vi "数组拆分.vi"(10 "拆分大小":i32=1000, 11 "输入数据":string[][](array[string])) -> (3 "输出数组":string[][](array[string]))   [LabVIEW 2016, in "数据传输系统-03.lvlib"]
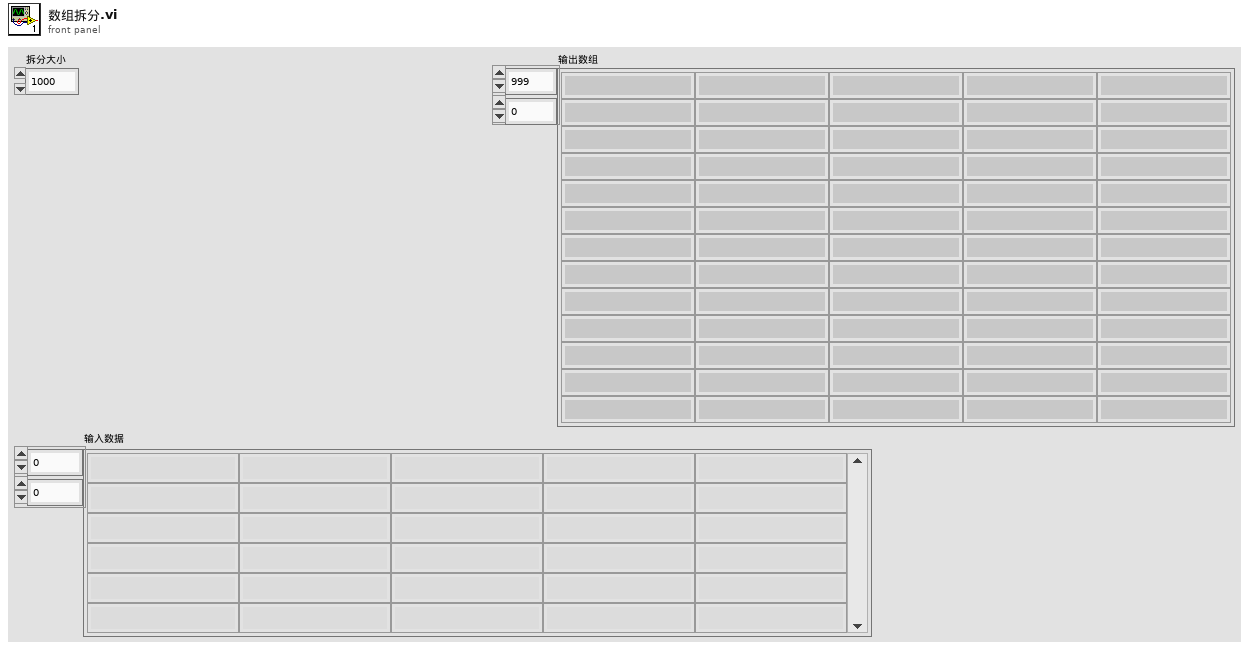
[diagram p1: front panel]
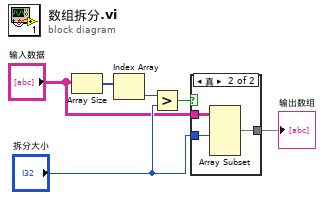
[diagram p0: block diagram]
diagram:
  n1 = Array Size(array="输入数据") -> (size(s)=w6:i32[])
  n2 = Index Array(array=w6) -> (element=w5:i32)  [unwired: 1 in]
  n3 = Greater?(x=w5, y="拆分大小") -> (0:w4:bool)
  n4 = case shown="真" w4 {
    tunnel: "输入数据" -> [w7 w10]
    tunnel: "拆分大小" -> [_ w9]
    tunnel: [w7 w8] -> w1
    frame False {
    }
    frame True {
      n5 = Array Subset(array=w10, length (row)=w9) -> (w8:string[][])  [unwired: 3 in]
    }
  }
  "输出数组" <- w1
